vi "Index.vi"(9 "Shoot2":bool, 10 "Shoot":bool, 11 "Output":dbl=-0.007874015748031496 format="%#_13g") -> ()   [LabVIEW 2016]
panel:
  in  "Max Effort":dbl=0.5 format="%#_13g"
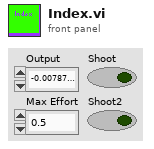
[diagram p1: front panel]
types:
  T1 = typedef "WPI_MotorControlDeviceRef.ctl" = cluster{"DeviceStatus":errorcluster, "Type":T2, "PWM":cluster{"PWM Channel":T3, "DeadBand":T4}, "CAN":cluster{"Device Number":u8, "SetOutput VI Ref":variant, "GetOutput VI Ref":variant, "Enable VI Ref":variant, "Disable VI Ref":variant, "Data":variant}, "Invert":bool}
  T2 = typedef "WPI_MotorControlType.ctl" = enum16{"PWM", "CAN"}
  T3 = typedef "FPGA_DIOPWMChannel.ctl" = enum8{"PWM 0", "PWM 1", "PWM 2", "PWM 3", "PWM 4", "PWM 5", "PWM 6", "PWM 7", "PWM 8", "PWM 9", "PWM MXP 0", "PWM MXP 1", "PWM MXP 2", "PWM MXP 3", "PWM MXP 4", "PWM MXP 5", "PWM MXP 6", "PWM MXP 7", "PWM MXP 8", "PWM MXP 9", "Invalid"}
  T4 = typedef "WPI_PWMDeadband.ctl" = cluster{"Name":string, "maxPositivePwm":i32, "minPositivePwm":i32, "centerPwm":i32, "maxNegativePwm":i32, "minNegativePwm":i32, "angularRange":u16}
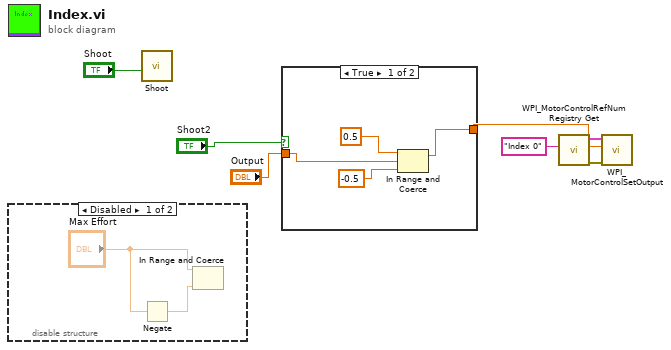
[diagram p0: block diagram]
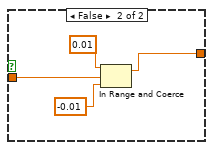
[diagram p3: hidden frame]
diagram:
  n1 = disable-structure shown="Disabled" {
    frame Disabled {
      n2 = Negate(x="Max Effort") -> (-x=w9:dbl)
      n3 = In Range and Coerce(upper limit="Max Effort", lower limit=w9) -> ()  [unwired: 1 in, 2 out]
    }
    frame Enabled {
    }
  }
  n4 = call "Shoot.vi"("Shoot"="Shoot") -> ()  [unwired: 10 in]
  n5 = case shown="True" "Shoot2" {
    tunnel: [w10 w15] -> w4
    tunnel: "Output" -> [w13 w14]
    frame True {
      n6 = In Range and Coerce(upper limit=0.5, x=w13, lower limit=-0.5 ("upper limit")) -> (coerced(x)=w10:dbl)  [unwired: 1 out]
    }
    frame False {
      n7 = In Range and Coerce(upper limit=0.01, x=w14, lower limit=-0.01 ("upper limit")) -> (coerced(x)=w15:dbl)  [unwired: 1 out]
    }
  }
  n8 = call <vilib>:"WPI_MotorControlRefNum Registry Get.vi"("refnum name"="Index 0") -> ("error out"=w6:errorcluster, "MotorControlDevRef"=w7:T1)  [unwired: 9 in]
  n9 = call <vilib>:"WPI_MotorControlSetOutput.vi"("error in (no error)"=w6, "Output"=w4, "MotorControlDevRef"=w7) -> ()  [unwired: 6 in, 3 out]
